vi "Command Drive Distance Slow.vi"(8 "Timeout":dbl=2.0, 9 "Heading":dbl=50.0, 10 "Distance":dbl=42.0, 11 "Startup":bool) -> (0 "Right Wheel":dbl, 1 "Reinit":bool, 2 "Left Wheel":dbl, 3 "Completed":bool=TRUE)   [LabVIEW 2017]
uses:
  Utility VIs/Refnum Names.vi
  Drive/Drive Globals.vi
panel:
  in  "Turn Gain":dbl=0.06
  in  "Gain":dbl=0.028
  # ".028"
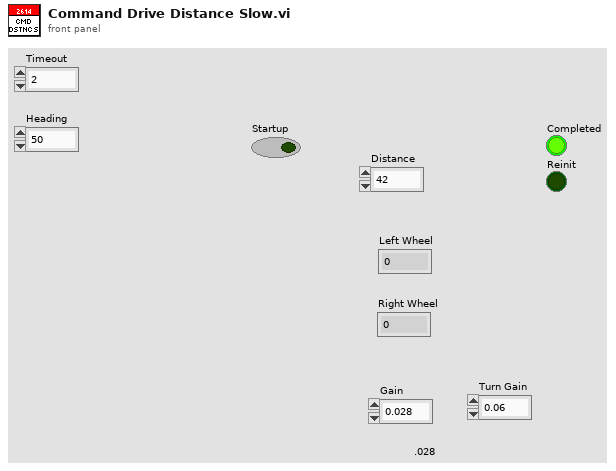
[diagram p1: front panel]
types:
  T1 = typedef "WPI_MotorControlDeviceRef.ctl" = cluster{"DeviceStatus":errorcluster, "Type":T2, "PWM":cluster{"PWM Channel":T3, "DeadBand":T4}, "CAN":cluster{"Device Number":u8, "SetOutput VI Ref":variant, "GetOutput VI Ref":variant, "Enable VI Ref":variant, "Disable VI Ref":variant, "Data":variant}, "Invert":bool, "DIO PWM":cluster{"PWM \"Enable\" Channel":T3, "DIOChannel":T5, "PWM Rate":dbl}}
  T2 = typedef "WPI_MotorControlType.ctl" = enum16{"PWM", "CAN", "DIO PWM"}
  T3 = typedef "FPGA_DIOPWMChannel.ctl" = enum8{"PWM 0", "PWM 1", "PWM 2", "PWM 3", "PWM 4", "PWM 5", "PWM 6", "PWM 7", "PWM 8", "PWM 9", "PWM MXP 0", "PWM MXP 1", "PWM MXP 2", "PWM MXP 3", "PWM MXP 4", "PWM MXP 5", "PWM MXP 6", "PWM MXP 7", "PWM MXP 8", "PWM MXP 9", "Invalid"}
  T4 = typedef "WPI_PWMDeadband.ctl" = cluster{"Name":string, "maxPositivePwm":i32, "minPositivePwm":i32, "centerPwm":i32, "maxNegativePwm":i32, "minNegativePwm":i32, "angularRange":u16}
  T5 = typedef "FPGA_DIOChannel.ctl" = enum8{"DIO 0", "DIO 1", "DIO 2", "DIO 3", "DIO 4", "DIO 5", "DIO 6", "DIO 7", "DIO 8", "DIO 9", "DIO MXP 0", "DIO MXP 1", "DIO MXP 2", "DIO MXP 3", "DIO MXP 4", "DIO MXP 5", "DIO MXP 6", "DIO MXP 7", "DIO MXP 8", "DIO MXP 9", "DIO MXP 10", "DIO MXP 11", "DIO MXP 12", "DIO MXP 13", "DIO MXP 14", "DIO MXP 15", "SPI Port CS1", "SPI Port CS2", "SPI Port CS3", "SPI Port MISO", "SPI Port MOSI", "Invalid"}
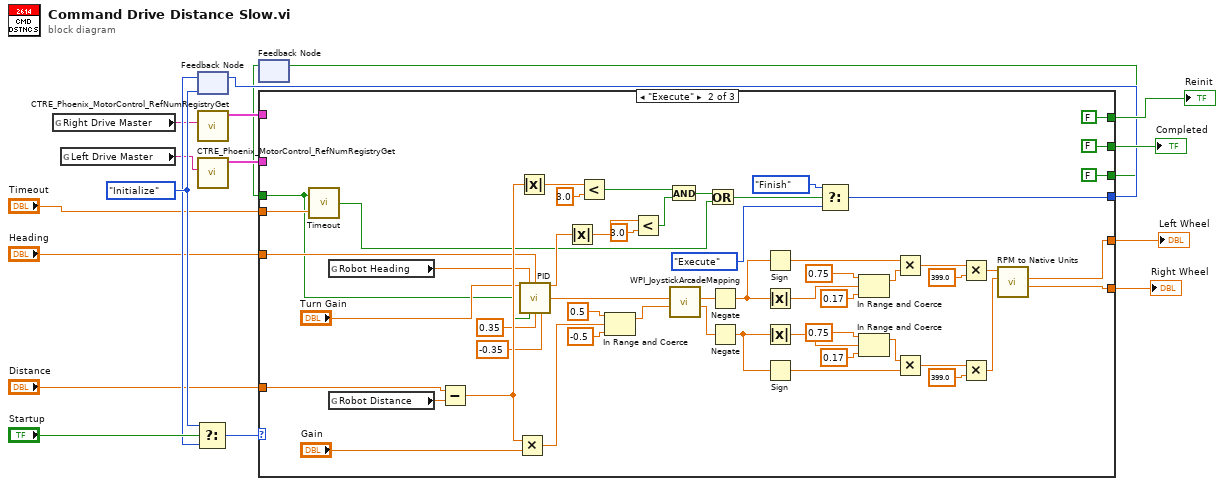
[diagram p0: block diagram]
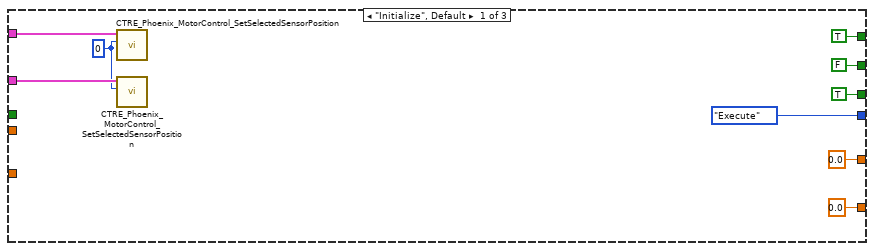
[diagram p2: hidden frame]
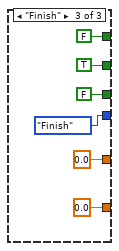
[diagram p3: hidden frame]
diagram:
  w16 = enum16{"Initialize", "Execute", "Finish"}."Initialize"
  n1 = global read "Refnum Names.vi" "Right Drive Master"() -> (w7:string)
  n2 = global read "Refnum Names.vi" "Left Drive Master"() -> (w8:string)
  n3 = feedback #1(w16) -> (w12:enum16{"Initialize", "Execute", "Finish"})
  n4 = Select(t=w16, s="Startup", f=w12) -> (s? t:f=w17:enum16{"Initialize", "Execute", "Finish"})
  n5 = call <vilib>:"CTRE_Phoenix_MotorControl_RefNumRegistryGet.vi"("refnum name"=w7) -> ("PhoenixMotorControlDevRef"=w6:T1)  [unwired: 9 in, 1 out]
  n6 = call <vilib>:"CTRE_Phoenix_MotorControl_RefNumRegistryGet.vi"("refnum name"=w8) -> ("PhoenixMotorControlDevRef"=w5:T1)  [unwired: 9 in, 1 out]
  n7 = feedback #2() -> (w2:bool)  [unwired: 1 in]
  n8 = case shown="\"Execute\"" w17 {
    tunnel: [FALSE FALSE TRUE] -> w15
    tunnel: [TRUE FALSE FALSE] -> w14
    tunnel: [enum16{"Initialize", "Execute", "Finish"}."Execute" w78 enum16{"Initialize", "Execute", "Finish"}."Finish"] -> w13
    tunnel: "Distance" -> [_ w77 _]
    tunnel: [0.0 ("Left Wheel Velocity") w31 0.0] -> w10
    tunnel: [0.0 ("Right Wheel Velocity") w30 0.0] -> w9
    tunnel: w6 -> [w21 _ _]
    tunnel: w5 -> [w22 _ _]
    tunnel: "Heading" -> [_ w57 _]
    tunnel: [TRUE FALSE FALSE] -> w3
    tunnel: w2 -> [_ w28 _]
    tunnel: "Timeout" -> [_ w50 _]
    frame "Initialize", Default {
      w20 = 0
      n9 = call <vilib>:"CTRE_Phoenix_MotorControl_SetSelectedSensorPosition.vi"("New Sensor Position"=w20, "PhoenixMotorControlDevRef"=w21) -> ()  [unwired: 8 in, 2 out]
      n10 = call <vilib>:"CTRE_Phoenix_MotorControl_SetSelectedSensorPosition.vi"("New Sensor Position"=w20, "PhoenixMotorControlDevRef"=w22) -> ()  [unwired: 8 in, 2 out]
    }
    frame "Execute" {
      n11 = call "Timeout.vi"("Timeout"=w50, "Initialize"=w28) -> ("Timed Out?"=w48:bool)
      n12 = global read "Drive Globals.vi" "Robot Heading"() -> (w71:dbl)
      n13 = global read "Drive Globals.vi" "Robot Distance"() -> (w76:dbl)
      n14 = Subtract(x=w77, y=w76) -> (x-y=w73:dbl)
      n15 = Multiply(x=w73, y="Gain") -> (x*y=w69:dbl)
      n16 = Absolute Value(x=w73) -> (abs(x)=w74:dbl)
      n17 = call "PID.vi"("Kp"="Turn Gain", "Process Variable"=w71, "Goal"=w57, "Reinit"=w28, "Max Ouput"=0.35, "Min Output"=-0.35) -> ("Current Error"=w58:dbl, "Command"=w56:dbl)  [unwired: 7 in, 1 out]
      n18 = Absolute Value(x=w58) -> (abs(x)=w60:dbl)
      n19 = Less?(x=w74, y=3.0) -> (x < y?=w62:bool)
      n20 = In Range and Coerce(upper limit=0.5, x=w69, lower limit=-0.5) -> (coerced(x)=w29:dbl)  [unwired: 1 out]
      n21 = Less?(x=w60, y=3.0) -> (x < y?=w59:bool)
      n22 = And(x=w62, y=w59) -> (x .and. y?=w63:bool)
      n23 = call <vilib>:"WPI_JoystickArcadeMapping.vi"("Y axis value"=w29, "X axis value"=w56) -> ("Right Motor Value"=w54:dbl, "Left Motor Value"=w55:dbl)  [unwired: 8 in]
      n24 = Or(x=w63, y=w48) -> (x .or. y?=w49:bool)
      n25 = Negate(x=w55) -> (-x=w44:dbl)
      n26 = Negate(x=w54) -> (-x=w45:dbl)
      n27 = Sign(1:w44) -> (0:w43:dbl)
      n28 = Absolute Value(x=w44) -> (abs(x)=w47:dbl)
      n29 = Absolute Value(x=w45) -> (abs(x)=w46:dbl)
      n30 = Sign(1:w45) -> (0:w38:dbl)
      n31 = Select(t=enum16{"Initialize", "Execute", "Finish"}."Finish", s=w49, f=enum16{"Initialize", "Execute", "Finish"}."Execute") -> (s? t:f=w78:enum16{"Initialize", "Execute", "Finish"})
      n32 = In Range and Coerce(upper limit=0.75, x=w47, lower limit=0.17) -> (coerced(x)=w42:dbl)  [unwired: 1 out]
      n33 = In Range and Coerce(upper limit=0.75, x=w46, lower limit=0.17) -> (coerced(x)=w39:dbl)  [unwired: 1 out]
      n34 = Multiply(x=w43, y=w42) -> (x*y=w41:dbl)
      n35 = Multiply(x=w39, y=w38) -> (x*y=w40:dbl)
      n36 = Multiply(x=w41, y=399.0) -> (x*y=w33:dbl)
      n37 = Multiply(x=w40, y=399.0) -> (x*y=w32:dbl)
      n38 = call "RPM to Native Units.vi"("Right RPM"=w32, "Left RPM"=w33) -> ("Right Out"=w30:dbl, "Left Out"=w31:dbl)  [unwired: 6 in, 1 out]
    }
    frame "Finish" {
    }
  }
  "Completed" <- w15
  "Reinit" <- w14
  "Left Wheel" <- w10
  "Right Wheel" <- w9
  n39 = feedback-in #1(w13) -> ()
  n40 = feedback-in #2(w3) -> ()
